vi "RecipeEditor_TestUI.vi"(8 "error in (no error)":errorcluster) -> (0 "error out":errorcluster)   [LabVIEW 2018]
panel:
  in  "Loaded":bool
  in  "Select Base Script":path
  in  "MZ Target":dbl=25000.0
  in  "MZ End":dbl=100000.0
  in  "MZ Start":dbl=15000.0
  in  "Aux Amp":ext=0.999999999 format="%#.8g"
  in  "MZ Aux Scan Stop":dbl=40000.0
  in  "MZ Aux Scan Start":dbl=25000.0
  in  "Laser Shots":dbl=3.0
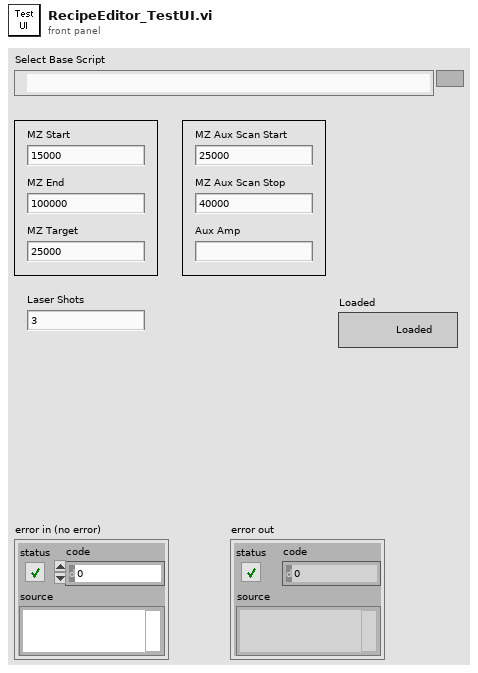
[diagram p1: front panel]
types:
  T1 = cluster{"MZ Start":dbl, "MZ End":dbl, "MZ Target":dbl, "Laser Shots":dbl, "MZ Aux Scan Start":dbl, "MZ Aux Scan Stop":dbl, "Aux Amp":ext}
  T2 = enum16{"open", "replace", "create", "open or create", "replace or create", "replace or create with confirmation"}
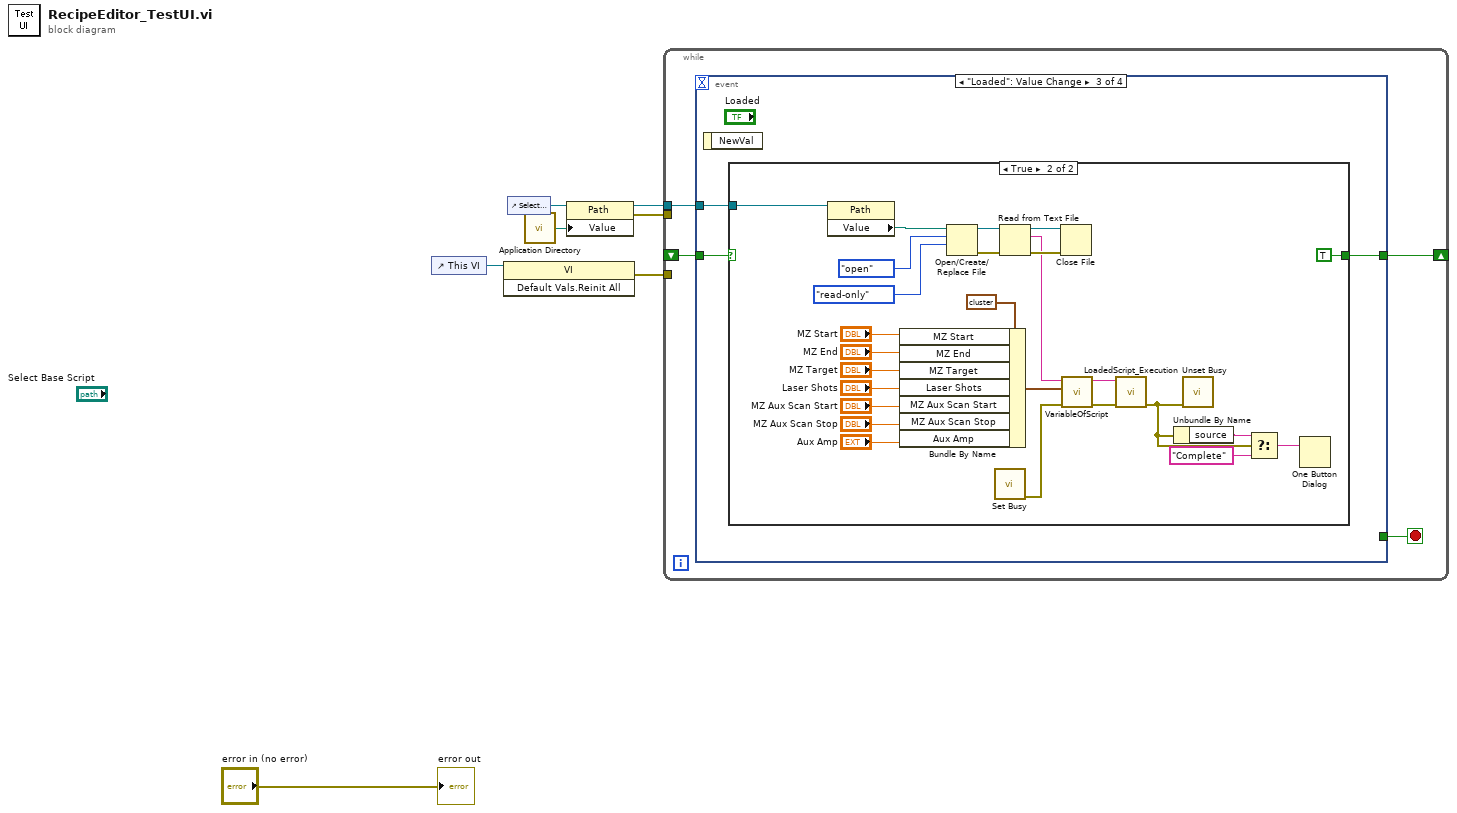
[diagram p0: block diagram]
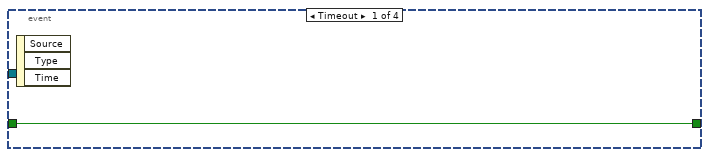
[diagram p2: hidden frame]
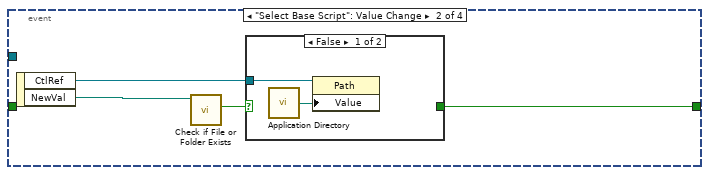
[diagram p3: hidden frame]
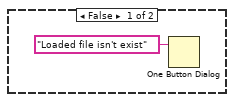
[diagram p5: hidden frame]
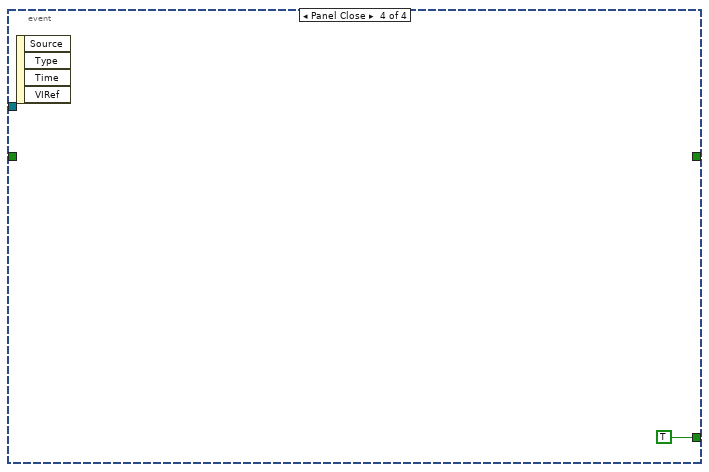
[diagram p6: hidden frame]
diagram:
  n1 = control-ref of="This VI"() -> (w4:refnum<vi>)
  n2 = invoke class="VI" method="Default Vals.Reinit All"(reference=w4) -> (error out=w3:errorcluster)  [unwired: 2 in, 2 out]
  n3 = control-ref of="Select Base Script"() -> (w7:refnum<vi>)
  n4 = call <vilib>:"Application Directory.vi"() -> ("Application Directory"=w6:path)
  n5 = property class="Path"(reference=w7, "Value"=w6) -> (reference out=w2:refnum<vi>, error out=w5:errorcluster)  [unwired: 1 in]
  n6 = while {
    tunnel: w5 -> [_]
    tunnel: w3 -> [_]
    tunnel: w2 -> [w11]
    shift-right: [w10] -> _
    shift-left: _ -> [w9]
    stop <- w8 stop-if-true
    n7 = event shown="[2] \"Loaded\": Value Change" {
      selector: _ -> [_ _ _ _]
      dyn-events: _ -> [_ _ _ _]
      timeout: _ -> [_ _ _ _]
      tunnel: w11 -> [_ _ w21 _]
      tunnel: [w12 w13 w20 _] -> w10
      tunnel: w9 -> [w12 _ w22 _]
      tunnel: [_ _ _ TRUE] -> w8
      event Timeout {
        n8 = event-data() -> ()  [unwired: 1 in, 3 out]
      }
      event "Select Base Script": Value Change {
        n9 = event-data() -> ("CtlRef"=w15:refnum<vi>, "NewVal"=w16:path)  [unwired: 1 in]
        n10 = call <vilib>:"Check if File or Folder Exists.vi"("path"=w16) -> ("file or folder exists?"=w14:bool)  [unwired: 8 in, 2 out]
        n11 = case shown="False" w14 {
          selector: w14 -> [_ w19]
          tunnel: w15 -> [w18 _]
          tunnel: [_ w19] -> w13
          frame False {
            n12 = call <vilib>:"Application Directory.vi"() -> ("Application Directory"=w17:path)
            n13 = property class="Path"(reference=w18, "Value"=w17) -> ()  [unwired: 1 in, 2 out]
          }
          frame True {
          }
        }
      }
      event "Loaded": Value Change {
        n14 = event-data() -> ()  [unwired: 1 in, 1 out]
        n15 = case shown="True" w22 {
          tunnel: w21 -> [_ w43]
          tunnel: [_ TRUE] -> w20
          frame False {
            n16 = One Button Dialog(message="Loaded file isn't exist") -> ()  [unwired: 1 in, 1 out]
          }
          frame True {
            n17 = property class="Path"(reference=w43) -> ("Value"=w42:path)  [unwired: 1 in, 2 out]
            n18 = Bundle By Name(cluster=T1 {"MZ Start"=15000.0, "MZ End"=100000.0, "MZ Target"=25000.0, "Laser Shots"=3.0, "MZ Aux Scan Start"=25000.0, "MZ Aux Scan Stop"=40000.0, "Aux Amp"=1.0}, "MZ Start"="MZ Start", "MZ End"="MZ End", "MZ Target"="MZ Target", "Laser Shots"="Laser Shots", "MZ Aux Scan Start"="MZ Aux Scan Start", "MZ Aux Scan Stop"="MZ Aux Scan Stop", "Aux Amp"="Aux Amp") -> (w32:T1)
            n19 = Open/Create/Replace File(file path (use dialog)=w42, operation (0:open)=T2."open", access (0:read/write)=enum16{"read/write", "read-only", "write-only"}."read-only") -> (refnum out=w44:refnum<file>, error out=w45:errorcluster)  [unwired: 3 in, 1 out]
            n20 = call <vilib>:"Set Busy.vi"() -> ("error out"=w29:errorcluster)  [unwired: 10 in, 1 out]
            n21 = Read from Text File(file (use dialog)=w44, error in=w45) -> (refnum out=w48:refnum<file>, text=w33:string, error out=w49:errorcluster)  [unwired: 2 in, 1 out]
            n22 = Close File(refnum=w48, error in=w49) -> ()  [unwired: 2 out]
            n23 = call "VariableOfScript.vi"("error in (no error)"=w29, "Cluster"=w32, "RawScripeString"=w33) -> ("error out"=w30:errorcluster, "RawScripeString Output"=w31:string)  [unwired: 7 in]
            n24 = call "LoadedScript_Execution.vi"("error in (no error)"=w30, "Script of MS Process"=w31) -> ("error out"=w27:errorcluster)  [unwired: 9 in]
            n25 = Unbundle By Name(w27) -> ("source"=w26:string)
            n26 = call <vilib>:"Unset Busy.vi"("error in (no error)"=w27) -> ()  [unwired: 10 in, 1 out]
            n27 = Select(t=w26, s=w27, f="Complete") -> (s? t:f=w24:string)
            n28 = One Button Dialog(message=w24) -> ()  [unwired: 1 in, 1 out]
          }
        }
      }
      event Panel Close {
        n29 = event-data() -> ()  [unwired: 1 in, 4 out]
      }
    }
  }
  "error out" <- "error in (no error)"
